vi "TX_TCP_Module.vi"(8 "error out":errorcluster, 10 "Event Registration Refnum":refnum<event-registration>, 11 "queue out":refnum<queue>) -> (0 "error out 2":errorcluster)   [LabVIEW 2023]
uses:
  TX_Control 3.ctl
  <vilib>/vision/Image Controls.llb/IMAQ Image.ctl
  TX_Cluster1TypeDef.ctl
  <vilib>/vision/NI_Vision_Development_Module.lvlib
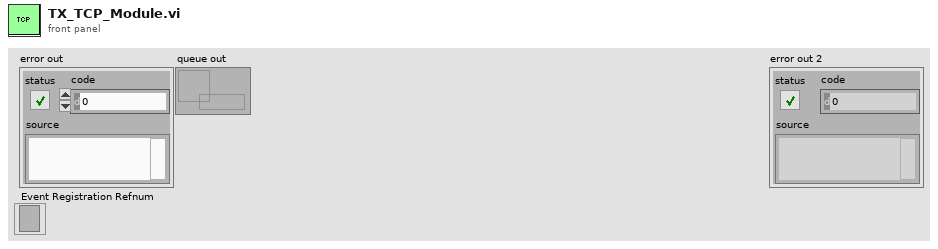
[diagram p1: front panel]
types:
  T1 = typedef "TX_Cluster1TypeDef.ctl" = cluster{"Enum":T2, "CamSel":variant, "CamView":variant}
  T2 = typedef "TX_Control 3.ctl" = enum16{"Default", "StartCamera", "TakePhoto", "EnableTCP", "Cam2Display", "CloseAll"}
  T3 = typedef "IMAQ Image.ctl" = refnum<image>
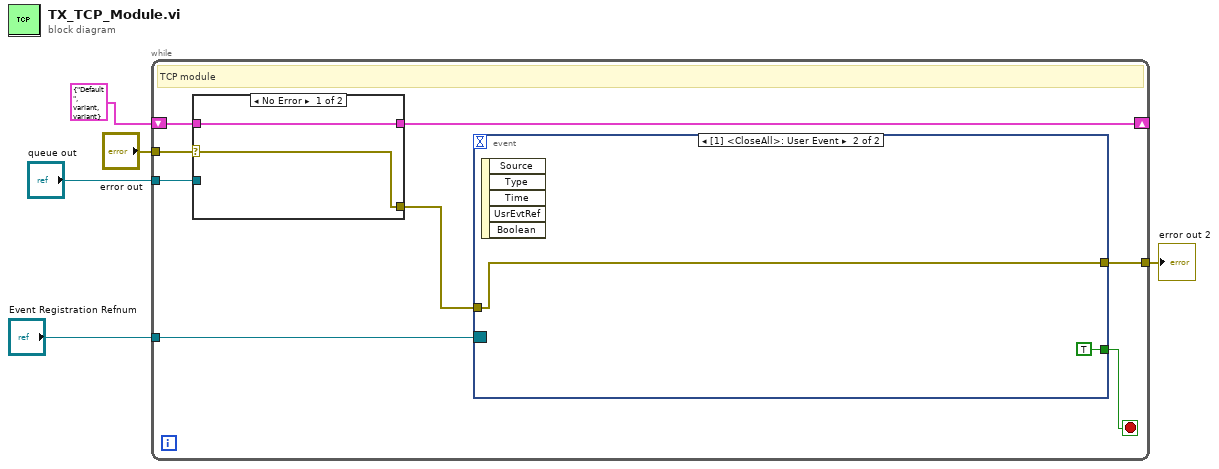
[diagram p0: block diagram]
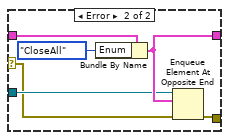
[diagram p2: hidden frame]
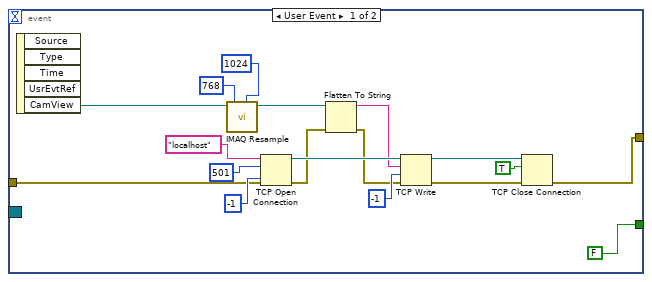
[diagram p3: hidden frame]
diagram:
  n1 = while {
    tunnel: "Event Registration Refnum" -> [w12]
    tunnel: [w11] -> w1
    tunnel: "error out" -> [w10]
    shift-right: [w8] -> _
    shift-left: T1 {"Enum"=enum."Default", "CamSel"=variant(refnum<image> refnum), "CamView"=variant(refnum<image> refnum)} ("Cluster") -> [w9]
    tunnel: "queue out" -> [w7]
    stop <- w13 stop-if-true
    # "TCP module"
    n2 = case shown="No Error" w10 {
      selector: w10 -> [w14 w17]
      tunnel: [w15 w19] -> w8
      tunnel: w9 -> [w15 w21]
      tunnel: w7 -> [_ w18]
      tunnel: [w14 w16] -> w6
      frame No Error {
      }
      frame Error {
        n3 = Bundle By Name(cluster=w21, "Enum"=TX_Control_3."CloseAll") -> (w19:T1)
        n4 = Enqueue Element At Opposite End(queue=w18, element=w19, error in (no error)=w17) -> (error out=w16:errorcluster)  [unwired: 1 in, 2 out]
      }
    }
    n5 = event shown="[1] <CloseAll>: User Event" {
      selector: w12 -> [_ _]
      dyn-events: _ -> [_ _]
      timeout: _ -> [_ _]
      tunnel: [FALSE TRUE] -> w13
      tunnel: [w31 w40] -> w11
      tunnel: w6 -> [w24 w40]
      event User Event {
        n6 = event-data() -> ("CamView"=w27:T3)  [unwired: 1 in, 4 out]
        n7 = call "IMAQ Resample"("X Resolution"=1024, "Y Resolution"=768, "Image Src"=w27) -> ("Image Dst Out"=w25:T3)  [unwired: 7 in, 1 out]
        n8 = TCP Open Connection(address="localhost", remote port or service name=u16 501, timeout ms (60000)=-1, error in (no error)=w24) -> (connection ID=w32:refnum<k5>, error out=w23:errorcluster)  [unwired: 1 in]
        n9 = Flatten To String(anything=w25, error in (no error)=w23) -> (data string=w26:string, error out=w22:errorcluster)  [unwired: 2 in, 1 out]
        n10 = TCP Write(connection ID=w32, data in=w26, error in (no error)=w22, 9:-1 ("timeout ms (25000)")) -> (connection ID out=w29:refnum<k5>, error out=w30:errorcluster)  [unwired: 1 out]
        n11 = TCP Close Connection(connection ID=w29, abort (F)=TRUE, error in (no error)=w30) -> (error out=w31:errorcluster)  [unwired: 1 out]
      }
      event User Event {
        n12 = event-data() -> ()  [unwired: 1 in, 5 out]
      }
    }
  }
  "error out 2" <- w1
